vi "URI Encode String.vi"(9 "Encode /":bool=TRUE, 11 "Un-encoded String":string) -> (3 "UriEncoded String":string)   [LabVIEW 2015, in "NI_Azure_Core.lvlib"]
uses:
  NI_Azure_Core.lvlib
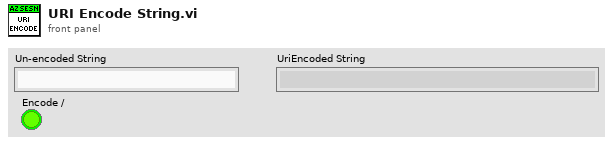
[diagram p1: front panel]
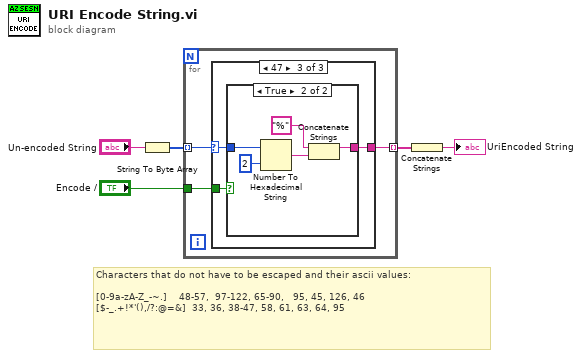
[diagram p0: block diagram]
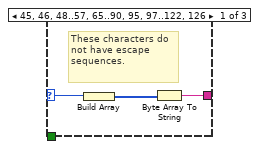
[diagram p2: hidden frame]
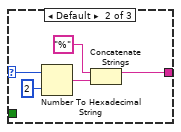
[diagram p3: hidden frame]
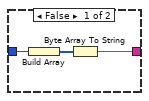
[diagram p4: hidden frame]
diagram:
  # "Characters that do not have to be escaped and their ascii values:\n\n[0-9a-zA-Z_-~.]    48-57,  97-122, 65-90,   95, 45, 126, 46 \n[$-_.+!*'(),/?:@=&]  33, 36, 38-47, 58, 61, 63, 64, 95"
  n1 = String To Byte Array(string="Un-encoded String") -> (unsigned byte array=w5:u8[])
  n2 = for {
    tunnel: w5 -> [w8] mode=indexing
    tunnel: "Encode /" -> [w7]
    tunnel: [w6] -> w2 mode=indexing
    n3 = case shown="47" w8 {
      selector: w8 -> [w11 w14 w19]
      tunnel: [w9 w13 w18] -> w6
      tunnel: w7 -> [_ _ w17]
      frame 45, 46, 48..57, 65..90, 95, 97..122, 126 {
        # "These characters do not have escape sequences."
        n4 = Build Array(w11) -> (w10:u8[])
        n5 = Byte Array To String(unsigned byte array=w10) -> (string=w9:string)
      }
      frame Default {
        n6 = Number To Hexadecimal String(1:i16 2 ("width (-)"), 2:w14) -> (0:w15:string)
        n7 = Concatenate Strings("%" ("string"), w15) -> (w13:string)
      }
      frame 47 {
        n8 = case shown="True" w17 {
          tunnel: w19 -> [w21 w23]
          tunnel: [w20 w25] -> w18
          frame False {
            n9 = Build Array(w21) -> (w22:u8[])
            n10 = Byte Array To String(unsigned byte array=w22) -> (string=w20:string)
          }
          frame True {
            n11 = Number To Hexadecimal String(1:i16 2 ("width (-)"), 2:w23) -> (0:w26:string)
            n12 = Concatenate Strings("%" ("string"), w26) -> (w25:string)
          }
        }
      }
    }
  }
  n13 = Concatenate Strings(w2) -> (→"UriEncoded String":string)
